vi "LabVIEW_MQTT_Toolkit_V2.vi"() -> ()   [LabVIEW 2021] (continued)
                  n1492 = Format Date/Time String(seconds (now)=w3662, UTC format=TRUE) -> (date/time string=w3664:string)  [unwired: 1 in]
                  n1493 = Build Array(w3677, w3680) -> (w3679:string[])
                  n1494 = Scan From String(format string="%<%x %H:%M:%S%3u>T", input string=w3664) -> (output 1=w3665:timestamp)  [unwired: 3 in, 3 out]
                  n1495 = To Double Precision Float(number=w3665) -> (double precision float=w3663:dbl)
                }
                n1496 = Concatenate Strings(w3623, "TimeStamp;MeasureCh_Z(g);", "\n") -> (w3639:string)
                n1497 = Build Path(base path=w3640, name or relative path="Logfile") -> (appended path=w3641:path)
                n1498 = Search and Replace String(replace all?=TRUE ("replace all? (F)"), input string=w3634, search string="/") -> (result string=w3646:string)  [unwired: 5 in, 3 out]
                n1499 = call <vilib>:"Check if File or Folder Exists.vi"("path"=w3641) -> ("file or folder exists?"=w3642:bool, "dup path"=w3643:path)  [unwired: 8 in, 1 out]
                n1500 = case shown="False" w3642 {
                  tunnel: w3643 -> [w3660 w3661]
                  tunnel: [w3659 w3661] -> w3644
                  frame False {
                    n1501 = Create Folder(path (use dialog)=w3660) -> (created path=w3659:path)  [unwired: 2 in, 2 out]
                  }
                  frame True {
                  }
                }
                n1502 = Concatenate Strings(w3646, "_" ("string"), "S_E_T.csv") -> (w3647:string)
                n1503 = Build Path(base path=w3644, name or relative path=w3647) -> (appended path=w3645:path)
                n1504 = Open/Create/Replace File(file path (use dialog)=w3645, operation (0:open)=T11."open or create") -> (refnum out=w3638:refnum<file>, error out=w3636:errorcluster)  [unwired: 4 in, 1 out]
                n1505 = Write to Text File(file (use dialog)=w3638, text=w3639, error in=w3636) -> (refnum out=w3637:refnum<file>, error out=w3635:errorcluster)  [unwired: 1 in, 1 out]
                n1506 = Close File(refnum=w3637, error in=w3635) -> (path=w3624:path)  [unwired: 1 out]
              }
              frame 2 {
                w3689 = T14 2 items=["User Home"=0, "User Desktop"=1, "User Documents"=2, "User Application Data"=3, "User Preferences"=4, "User Temporary"=5, "Public Documents"=6, "Public Application Data"=7, "Public Preferences"=8, "Public Cache"=13, "System Core Libraries"=9, "System Installed Libraries"=10, "Application Files"=11, "Boot Volume Root"=12] ("system directory type")
                n1507 = Decimate 1D Array(w3716) -> (w3714:dbl[])
                n1508 = Search and Replace String(replace all?=TRUE ("replace all? (F)"), input string=w3684, search string="/") -> (result string=w3705:string)  [unwired: 5 in, 3 out]
                n1509 = for {
                  tunnel: w3714 -> [w3735] mode=indexing
                  tunnel: [w3738] -> w3713 mode=indexing
                  tunnel: w3715 -> [w3737] mode=indexing
                  tunnel: [w3735] -> w3712 mode=indexing
                  tunnel: w3711 -> [w3730]
                  tunnel: w3710 -> [w3729]
                  tunnel: w3709 -> [w3728] mode=indexing
                  tunnel: w3708 -> [w3727]
                  tunnel: [w3722] -> w3707
                  n1510 = Join Numbers(hi=w3730, lo=w3729) -> ((hi.lo)=w3732:u32)
                  n1511 = To Double Precision Float(number=w3728) -> (double precision float=w3733:dbl)
                  n1512 = Number To Decimal String(number=w3737) -> (decimal integer string=w3736:string)  [unwired: 1 in]
                  n1513 = Number To Fractional String(number=w3735, precision (6)=i16 3 ("width (-)")) -> (F-format string=w3739:string)  [unwired: 2 in]
                  n1514 = Divide(x=w3733, y=w3727) -> (x/y=w3734:dbl)
                  n1515 = Build Array(w3736, w3739) -> (w3738:string[])
                  n1516 = To Unsigned Quad Integer(1:w3732) -> (0:w3731:u64)
                  n1517 = call "Unix Time to Timestamp.vi"("Fractional Second"=w3734, "Unix Time (s)"=w3731) -> ("Timestamp"=w3721:timestamp)  [unwired: 8 in, 1 out]
                  n1518 = Format Date/Time String(seconds (now)=w3721, UTC format=TRUE) -> (date/time string=w3723:string)  [unwired: 1 in]
                  n1519 = Scan From String(format string="%<%x %H:%M:%S%3u>T", input string=w3723) -> (output 1=w3724:timestamp)  [unwired: 3 in, 3 out]
                  n1520 = To Double Precision Float(number=w3724) -> (double precision float=w3722:dbl)
                }
                n1521 = Concatenate Strings(w3682, "TimeStamp;MeasureCh_X(g);", "\n") -> (w3698:string)
                n1522 = Concatenate Strings(w3705, "_" ("string"), "S_E_T.csv") -> (w3706:string)
                n1523 = call <vilib>:"Get System Directory.vi"("system directory type"=w3689) -> ("system directory"=w3699:path)  [unwired: 10 in]
                n1524 = Build Path(base path=w3699, name or relative path="Logfile") -> (appended path=w3700:path)
                n1525 = call <vilib>:"Check if File or Folder Exists.vi"("path"=w3700) -> ("file or folder exists?"=w3701:bool, "dup path"=w3702:path)  [unwired: 8 in, 1 out]
                n1526 = case shown="False" w3701 {
                  tunnel: w3702 -> [w3719 w3720]
                  tunnel: [w3718 w3720] -> w3703
                  frame False {
                    n1527 = Create Folder(path (use dialog)=w3719) -> (created path=w3718:path)  [unwired: 2 in, 2 out]
                  }
                  frame True {
                  }
                }
                n1528 = Build Path(base path=w3703, name or relative path=w3706) -> (appended path=w3704:path)
                n1529 = Open/Create/Replace File(file path (use dialog)=w3704, operation (0:open)=T11."open or create") -> (refnum out=w3697:refnum<file>, error out=w3695:errorcluster)  [unwired: 4 in, 1 out]
                n1530 = Write to Text File(file (use dialog)=w3697, text=w3698, error in=w3695) -> (refnum out=w3696:refnum<file>, error out=w3694:errorcluster)  [unwired: 1 in, 1 out]
                n1531 = Close File(refnum=w3696, error in=w3694) -> (path=w3683:path)  [unwired: 1 out]
              }
              frame 3 {
                w3748 = T14 2 items=["User Home"=0, "User Desktop"=1, "User Documents"=2, "User Application Data"=3, "User Preferences"=4, "User Temporary"=5, "Public Documents"=6, "Public Application Data"=7, "Public Preferences"=8, "Public Cache"=13, "System Core Libraries"=9, "System Installed Libraries"=10, "Application Files"=11, "Boot Volume Root"=12] ("system directory type")
                n1532 = Decimate 1D Array(w3777) -> (w3775:dbl[], w3774:dbl[])
                n1533 = Search and Replace String(replace all?=TRUE ("replace all? (F)"), input string=w3743, search string="/") -> (result string=w3764:string)  [unwired: 5 in, 3 out]
                n1534 = Concatenate Strings(w3741, "TimeStamp;MeasureCh_Z(g);Ch_X(g);", "\n") -> (w3757:string)
                n1535 = for {
                  tunnel: w3775 -> [w3797] mode=indexing
                  tunnel: w3774 -> [w3796] mode=indexing
                  tunnel: [w3800] -> w3773 mode=indexing
                  tunnel: w3776 -> [w3799] mode=indexing
                  tunnel: [w3797] -> w3772 mode=indexing
                  tunnel: [w3796] -> w3771 mode=indexing
                  tunnel: w3770 -> [w3791]
                  tunnel: w3769 -> [w3790]
                  tunnel: w3768 -> [w3789] mode=indexing
                  tunnel: w3767 -> [w3788]
                  tunnel: [w3783] -> w3766
                  n1536 = Join Numbers(hi=w3791, lo=w3790) -> ((hi.lo)=w3793:u32)
                  n1537 = To Double Precision Float(number=w3789) -> (double precision float=w3794:dbl)
                  n1538 = Number To Decimal String(number=w3799) -> (decimal integer string=w3798:string)  [unwired: 1 in]
                  n1539 = Number To Fractional String(number=w3797, precision (6)=i16 3 ("width (-)")) -> (F-format string=w3802:string)  [unwired: 2 in]
                  n1540 = Number To Fractional String(number=w3796, precision (6)=i16 3 ("width (-)")) -> (F-format string=w3801:string)  [unwired: 2 in]
                  n1541 = Divide(x=w3794, y=w3788) -> (x/y=w3795:dbl)
                  n1542 = Build Array(w3798, w3802, w3801) -> (w3800:string[])
                  n1543 = To Unsigned Quad Integer(1:w3793) -> (0:w3792:u64)
                  n1544 = call "Unix Time to Timestamp.vi"("Fractional Second"=w3795, "Unix Time (s)"=w3792) -> ("Timestamp"=w3782:timestamp)  [unwired: 8 in, 1 out]
                  n1545 = Format Date/Time String(seconds (now)=w3782, UTC format=TRUE) -> (date/time string=w3784:string)  [unwired: 1 in]
                  n1546 = Scan From String(format string="%<%x %H:%M:%S%3u>T", input string=w3784) -> (output 1=w3785:timestamp)  [unwired: 3 in, 3 out]
                  n1547 = To Double Precision Float(number=w3785) -> (double precision float=w3783:dbl)
                }
                n1548 = Concatenate Strings(w3764, "_" ("string"), "S_E_T.csv") -> (w3765:string)
                n1549 = call <vilib>:"Get System Directory.vi"("system directory type"=w3748) -> ("system directory"=w3758:path)  [unwired: 10 in]
                n1550 = Build Path(base path=w3758, name or relative path="Logfile") -> (appended path=w3759:path)
                n1551 = call <vilib>:"Check if File or Folder Exists.vi"("path"=w3759) -> ("file or folder exists?"=w3760:bool, "dup path"=w3761:path)  [unwired: 8 in, 1 out]
                n1552 = case shown="False" w3760 {
                  tunnel: w3761 -> [w3780 w3781]
                  tunnel: [w3779 w3781] -> w3762
                  frame False {
                    n1553 = Create Folder(path (use dialog)=w3780) -> (created path=w3779:path)  [unwired: 2 in, 2 out]
                  }
                  frame True {
                  }
                }
                n1554 = Build Path(base path=w3762, name or relative path=w3765) -> (appended path=w3763:path)
                n1555 = Open/Create/Replace File(file path (use dialog)=w3763, operation (0:open)=T11."open or create") -> (refnum out=w3756:refnum<file>, error out=w3754:errorcluster)  [unwired: 4 in, 1 out]
                n1556 = Write to Text File(file (use dialog)=w3756, text=w3757, error in=w3754) -> (refnum out=w3755:refnum<file>, error out=w3753:errorcluster)  [unwired: 1 in, 1 out]
                n1557 = Close File(refnum=w3755, error in=w3753) -> (path=w3742:path)  [unwired: 1 out]
              }
              frame 4 {
                w3812 = T14 2 items=["User Home"=0, "User Desktop"=1, "User Documents"=2, "User Application Data"=3, "User Preferences"=4, "User Temporary"=5, "Public Documents"=6, "Public Application Data"=7, "Public Preferences"=8, "Public Cache"=13, "System Core Libraries"=9, "System Installed Libraries"=10, "Application Files"=11, "Boot Volume Root"=12] ("system directory type")
                # "this function calculate Time  of subpacket"
                n1558 = Decimate 1D Array(w3839) -> (w3838:dbl[])
                n1559 = Search and Replace String(replace all?=TRUE ("replace all? (F)"), input string=w3807, search string="/") -> (result string=w3828:string)  [unwired: 5 in, 3 out]
                n1560 = Concatenate Strings(w3805, "TimeStamp;MeasureCh_Y(g);", "\n") -> (w3821:string)
                n1561 = for {
                  tunnel: w3838 -> [w3858] mode=indexing
                  tunnel: [w3861] -> w3836 mode=indexing
                  tunnel: w3837 -> [w3860] mode=indexing
                  tunnel: [w3858] -> w3835 mode=indexing
                  tunnel: w3834 -> [w3853]
                  tunnel: w3833 -> [w3850]
                  tunnel: w3832 -> [w3851] mode=indexing
                  tunnel: w3831 -> [w3852]
                  tunnel: [w3844] -> w3830
                  n1562 = Join Numbers(hi=w3853, lo=w3850) -> ((hi.lo)=w3855:u32)
                  n1563 = To Double Precision Float(number=w3851) -> (double precision float=w3856:dbl)
                  n1564 = Number To Decimal String(number=w3860) -> (decimal integer string=w3859:string)  [unwired: 1 in]
                  n1565 = Number To Fractional String(number=w3858, precision (6)=i16 3 ("width (-)")) -> (F-format string=w3862:string)  [unwired: 2 in]
                  n1566 = Divide(x=w3856, y=w3852) -> (x/y=w3857:dbl)
                  n1567 = Build Array(w3859, w3862) -> (w3861:string[])
                  n1568 = To Unsigned Quad Integer(1:w3855) -> (0:w3854:u64)
                  n1569 = call "Unix Time to Timestamp.vi"("Fractional Second"=w3857, "Unix Time (s)"=w3854) -> ("Timestamp"=w3845:timestamp)  [unwired: 8 in, 1 out]
                  n1570 = Format Date/Time String(seconds (now)=w3845, UTC format=TRUE) -> (date/time string=w3846:string)  [unwired: 1 in]
                  n1571 = Scan From String(format string="%<%x %H:%M:%S%3u>T", input string=w3846) -> (output 1=w3847:timestamp)  [unwired: 3 in, 3 out]
                  n1572 = To Double Precision Float(number=w3847) -> (double precision float=w3844:dbl)
                }
                n1573 = Concatenate Strings(w3828, "_" ("string"), "S_E_T.csv") -> (w3829:string)
                n1574 = call <vilib>:"Get System Directory.vi"("system directory type"=w3812) -> ("system directory"=w3822:path)  [unwired: 10 in]
                n1575 = Build Path(base path=w3822, name or relative path="Logfile") -> (appended path=w3823:path)
                n1576 = call <vilib>:"Check if File or Folder Exists.vi"("path"=w3823) -> ("file or folder exists?"=w3824:bool, "dup path"=w3825:path)  [unwired: 8 in, 1 out]
                n1577 = case shown="False" w3824 {
                  tunnel: w3825 -> [w3842 w3843]
                  tunnel: [w3841 w3843] -> w3826
                  frame False {
                    n1578 = Create Folder(path (use dialog)=w3842) -> (created path=w3841:path)  [unwired: 2 in, 2 out]
                  }
                  frame True {
                  }
                }
                n1579 = Build Path(base path=w3826, name or relative path=w3829) -> (appended path=w3827:path)
                n1580 = Open/Create/Replace File(file path (use dialog)=w3827, operation (0:open)=T11."open or create") -> (refnum out=w3820:refnum<file>, error out=w3818:errorcluster)  [unwired: 4 in, 1 out]
                n1581 = Write to Text File(file (use dialog)=w3820, text=w3821, error in=w3818) -> (refnum out=w3819:refnum<file>, error out=w3817:errorcluster)  [unwired: 1 in, 1 out]
                n1582 = Close File(refnum=w3819, error in=w3817) -> (path=w3806:path)  [unwired: 1 out]
              }
              frame 5 {
                w3871 = T14 2 items=["User Home"=0, "User Desktop"=1, "User Documents"=2, "User Application Data"=3, "User Preferences"=4, "User Temporary"=5, "Public Documents"=6, "Public Application Data"=7, "Public Preferences"=8, "Public Cache"=13, "System Core Libraries"=9, "System Installed Libraries"=10, "Application Files"=11, "Boot Volume Root"=12] ("system directory type")
                n1583 = Decimate 1D Array(w3901) -> (w3897:dbl[], w3898:dbl[])
                n1584 = Search and Replace String(replace all?=TRUE ("replace all? (F)"), input string=w3865, search string="/") -> (result string=w3887:string)  [unwired: 5 in, 3 out]
                n1585 = for {
                  tunnel: [w3924] -> w3899 mode=indexing
                  tunnel: w3900 -> [w3923] mode=indexing
                  tunnel: w3897 -> [w3921] mode=indexing
                  tunnel: w3898 -> [w3920] mode=indexing
                  tunnel: [w3921] -> w3896 mode=indexing
                  tunnel: [w3920] -> w3895 mode=indexing
                  tunnel: w3894 -> [w3915]
                  tunnel: w3893 -> [w3914]
                  tunnel: w3892 -> [w3913] mode=indexing
                  tunnel: w3891 -> [w3912]
                  tunnel: [w3907] -> w3890
                  tunnel: [w3907] -> w3889
                  n1586 = Join Numbers(hi=w3915, lo=w3914) -> ((hi.lo)=w3917:u32)
                  n1587 = To Double Precision Float(number=w3913) -> (double precision float=w3918:dbl)
                  n1588 = Number To Decimal String(number=w3923) -> (decimal integer string=w3922:string)  [unwired: 1 in]
                  n1589 = Number To Fractional String(number=w3921, precision (6)=i16 3 ("width (-)")) -> (F-format string=w3926:string)  [unwired: 2 in]
                  n1590 = Number To Fractional String(number=w3920, precision (6)=i16 3 ("width (-)")) -> (F-format string=w3925:string)  [unwired: 2 in]
                  n1591 = Divide(x=w3918, y=w3912) -> (x/y=w3919:dbl)
                  n1592 = Build Array(w3922, w3926, w3925) -> (w3924:string[])
                  n1593 = To Unsigned Quad Integer(1:w3917) -> (0:w3916:u64)
                  n1594 = call "Unix Time to Timestamp.vi"("Fractional Second"=w3919, "Unix Time (s)"=w3916) -> ("Timestamp"=w3906:timestamp)  [unwired: 8 in, 1 out]
                  n1595 = Format Date/Time String(seconds (now)=w3906, UTC format=TRUE) -> (date/time string=w3908:string)  [unwired: 1 in]
                  n1596 = Scan From String(format string="%<%x %H:%M:%S%3u>T", input string=w3908) -> (output 1=w3909:timestamp)  [unwired: 3 in, 3 out]
                  n1597 = To Double Precision Float(number=w3909) -> (double precision float=w3907:dbl)
                }
                n1598 = Concatenate Strings(w3864, "TimeStamp;MeasureCh_Z(g);Ch_Y(g);", "\n") -> (w3880:string)
                n1599 = Concatenate Strings(w3887, "_" ("string"), "S_E_T.csv") -> (w3888:string)
                n1600 = call <vilib>:"Get System Directory.vi"("system directory type"=w3871) -> ("system directory"=w3881:path)  [unwired: 10 in]
                n1601 = Build Path(base path=w3881, name or relative path="Logfile") -> (appended path=w3882:path)
                n1602 = call <vilib>:"Check if File or Folder Exists.vi"("path"=w3882) -> ("file or folder exists?"=w3883:bool, "dup path"=w3884:path)  [unwired: 8 in, 1 out]
                n1603 = case shown="False" w3883 {
                  tunnel: w3884 -> [w3904 w3905]
                  tunnel: [w3903 w3905] -> w3885
                  frame False {
                    n1604 = Create Folder(path (use dialog)=w3904) -> (created path=w3903:path)  [unwired: 2 in, 2 out]
                  }
                  frame True {
                  }
                }
                n1605 = Build Path(base path=w3885, name or relative path=w3888) -> (appended path=w3886:path)
                n1606 = Open/Create/Replace File(file path (use dialog)=w3886, operation (0:open)=T11."open or create") -> (refnum out=w3879:refnum<file>, error out=w3877:errorcluster)  [unwired: 4 in, 1 out]
                n1607 = Write to Text File(file (use dialog)=w3879, text=w3880, error in=w3877) -> (refnum out=w3878:refnum<file>, error out=w3876:errorcluster)  [unwired: 1 in, 1 out]
                n1608 = Close File(refnum=w3878, error in=w3876) -> (path=w3866:path)  [unwired: 1 out]
              }
              frame 6 {
                w3936 = T14 2 items=["User Home"=0, "User Desktop"=1, "User Documents"=2, "User Application Data"=3, "User Preferences"=4, "User Temporary"=5, "Public Documents"=6, "Public Application Data"=7, "Public Preferences"=8, "Public Cache"=13, "System Core Libraries"=9, "System Installed Libraries"=10, "Application Files"=11, "Boot Volume Root"=12] ("system directory type")
                n1609 = Decimate 1D Array(w3966) -> (w3964:dbl[], w3963:dbl[])
                n1610 = Search and Replace String(replace all?=TRUE ("replace all? (F)"), input string=w3931, search string="/") -> (result string=w3952:string)  [unwired: 5 in, 3 out]
                n1611 = for {
                  tunnel: w3964 -> [w3986] mode=indexing
                  tunnel: w3963 -> [w3985] mode=indexing
                  tunnel: [w3989] -> w3962 mode=indexing
                  tunnel: w3965 -> [w3988] mode=indexing
                  tunnel: [w3986] -> w3961 mode=indexing
                  tunnel: [w3985] -> w3960 mode=indexing
                  tunnel: w3959 -> [w3980]
                  tunnel: w3958 -> [w3979]
                  tunnel: w3957 -> [w3978] mode=indexing
                  tunnel: w3956 -> [w3977]
                  tunnel: [w3972] -> w3955
                  tunnel: [w3972] -> w3954
                  n1612 = Join Numbers(hi=w3980, lo=w3979) -> ((hi.lo)=w3982:u32)
                  n1613 = To Double Precision Float(number=w3978) -> (double precision float=w3983:dbl)
                  n1614 = Number To Decimal String(number=w3988) -> (decimal integer string=w3987:string)  [unwired: 1 in]
                  n1615 = Number To Fractional String(number=w3986, precision (6)=i16 3 ("width (-)")) -> (F-format string=w3991:string)  [unwired: 2 in]
                  n1616 = Number To Fractional String(number=w3985, precision (6)=i16 3 ("width (-)")) -> (F-format string=w3990:string)  [unwired: 2 in]
                  n1617 = Divide(x=w3983, y=w3977) -> (x/y=w3984:dbl)
                  n1618 = Build Array(w3987, w3991, w3990) -> (w3989:string[])
                  n1619 = To Unsigned Quad Integer(1:w3982) -> (0:w3981:u64)
                  n1620 = call "Unix Time to Timestamp.vi"("Fractional Second"=w3984, "Unix Time (s)"=w3981) -> ("Timestamp"=w3971:timestamp)  [unwired: 8 in, 1 out]
                  n1621 = Format Date/Time String(seconds (now)=w3971, UTC format=TRUE) -> (date/time string=w3973:string)  [unwired: 1 in]
                  n1622 = Scan From String(format string="%<%x %H:%M:%S%3u>T", input string=w3973) -> (output 1=w3974:timestamp)  [unwired: 3 in, 3 out]
                  n1623 = To Double Precision Float(number=w3974) -> (double precision float=w3972:dbl)
                }
                n1624 = Concatenate Strings(w3930, "TimeStamp;MeasureCh_X(g);Ch_Y(g);", "\n") -> (w3945:string)
                n1625 = Concatenate Strings(w3952, "_" ("string"), "S_E_T.csv") -> (w3953:string)
                n1626 = call <vilib>:"Get System Directory.vi"("system directory type"=w3936) -> ("system directory"=w3946:path)  [unwired: 10 in]
                n1627 = Build Path(base path=w3946, name or relative path="Logfile") -> (appended path=w3947:path)
                n1628 = call <vilib>:"Check if File or Folder Exists.vi"("path"=w3947) -> ("file or folder exists?"=w3948:bool, "dup path"=w3949:path)  [unwired: 8 in, 1 out]
                n1629 = case shown="False" w3948 {
                  tunnel: w3949 -> [w3969 w3970]
                  tunnel: [w3968 w3970] -> w3950
                  frame False {
                    n1630 = Create Folder(path (use dialog)=w3969) -> (created path=w3968:path)  [unwired: 2 in, 2 out]
                  }
                  frame True {
                  }
                }
                n1631 = Build Path(base path=w3950, name or relative path=w3953) -> (appended path=w3951:path)
                n1632 = Open/Create/Replace File(file path (use dialog)=w3951, operation (0:open)=T11."open or create") -> (refnum out=w3944:refnum<file>, error out=w3942:errorcluster)  [unwired: 4 in, 1 out]
                n1633 = Write to Text File(file (use dialog)=w3944, text=w3945, error in=w3942) -> (refnum out=w3943:refnum<file>, error out=w3941:errorcluster)  [unwired: 1 in, 1 out]
                n1634 = Close File(refnum=w3943, error in=w3941) -> (path=w3929:path)  [unwired: 1 out]
              }
              frame 7 {
                w4001 = T14 2 items=["User Home"=0, "User Desktop"=1, "User Documents"=2, "User Application Data"=3, "User Preferences"=4, "User Temporary"=5, "Public Documents"=6, "Public Application Data"=7, "Public Preferences"=8, "Public Cache"=13, "System Core Libraries"=9, "System Installed Libraries"=10, "Application Files"=11, "Boot Volume Root"=12] ("system directory type")
                n1635 = Search and Replace String(replace all?=TRUE ("replace all? (F)"), input string=w3996, search string="/") -> (result string=w4017:string)  [unwired: 5 in, 3 out]
                n1636 = Concatenate Strings(w3994, "TimeStamp;MeasureCh_Z(g);Ch_X(g);Ch_Y(g);", "\n") -> (w4010:string)
                n1637 = Concatenate Strings(w4017, "_" ("string"), "S_E_T.csv") -> (w4018:string)
                n1638 = call <vilib>:"Get System Directory.vi"("system directory type"=w4001) -> ("system directory"=w4011:path)  [unwired: 10 in]
                n1639 = Decimate 1D Array(w4034) -> (w4033:dbl[], w4032:dbl[], w4031:dbl[])
                n1640 = for {
                  tunnel: w4033 -> [w4055] mode=indexing
                  tunnel: w4032 -> [w4054] mode=indexing
                  tunnel: w4031 -> [w4053] mode=indexing
                  tunnel: [w4058] -> w4030 mode=indexing
                  tunnel: w4029 -> [w4057] mode=indexing
                  tunnel: [w4055] -> w4028 mode=indexing
                  tunnel: [w4054] -> w4027 mode=indexing
                  tunnel: [w4053] -> w4026 mode=indexing
                  tunnel: w4025 -> [w4048]
                  tunnel: w4024 -> [w4047]
                  tunnel: w4023 -> [w4046] mode=indexing
                  tunnel: w4022 -> [w4045]
                  tunnel: [w4039] -> w4021
                  tunnel: [w4039] -> w4020
                  tunnel: [w4039] -> w4019
                  n1641 = Join Numbers(hi=w4048, lo=w4047) -> ((hi.lo)=w4050:u32)
                  n1642 = To Double Precision Float(number=w4046) -> (double precision float=w4051:dbl)
                  n1643 = Number To Decimal String(number=w4057) -> (decimal integer string=w4056:string)  [unwired: 1 in]
                  n1644 = Number To Fractional String(number=w4055, precision (6)=i16 3 ("width (-)")) -> (F-format string=w4062:string)  [unwired: 2 in]
                  n1645 = Number To Fractional String(number=w4054, precision (6)=i16 3 ("width (-)")) -> (F-format string=w4061:string)  [unwired: 2 in]
                  n1646 = Number To Fractional String(number=w4053, precision (6)=i16 3 ("width (-)")) -> (F-format string=w4059:string)  [unwired: 2 in]
                  n1647 = Build Array(w4056, w4062, w4061, w4059) -> (w4058:string[])
                  n1648 = Divide(x=w4051, y=w4045) -> (x/y=w4052:dbl)
                  n1649 = To Unsigned Quad Integer(1:w4050) -> (0:w4049:u64)
                  n1650 = call "Unix Time to Timestamp.vi"("Fractional Second"=w4052, "Unix Time (s)"=w4049) -> ("Timestamp"=w4040:timestamp)  [unwired: 8 in, 1 out]
                  n1651 = Format Date/Time String(seconds (now)=w4040, UTC format=TRUE) -> (date/time string=w4041:string)  [unwired: 1 in]
                  n1652 = Scan From String(format string="%<%x %H:%M:%S%3u>T", input string=w4041) -> (output 1=w4042:timestamp)  [unwired: 3 in, 3 out]
                  n1653 = To Double Precision Float(number=w4042) -> (double precision float=w4039:dbl)
                }
                n1654 = Build Path(base path=w4011, name or relative path="Logfile") -> (appended path=w4012:path)
                n1655 = call <vilib>:"Check if File or Folder Exists.vi"("path"=w4012) -> ("file or folder exists?"=w4013:bool, "dup path"=w4014:path)  [unwired: 8 in, 1 out]
                n1656 = case shown="False" w4013 {
                  tunnel: w4014 -> [w4037 w4038]
                  tunnel: [w4036 w4038] -> w4015
                  frame False {
                    n1657 = Create Folder(path (use dialog)=w4037) -> (created path=w4036:path)  [unwired: 2 in, 2 out]
                  }
                  frame True {
                  }
                }
                n1658 = Build Path(base path=w4015, name or relative path=w4018) -> (appended path=w4016:path)
                n1659 = Open/Create/Replace File(file path (use dialog)=w4016, operation (0:open)=T11."open or create") -> (refnum out=w4009:refnum<file>, error out=w4007:errorcluster)  [unwired: 4 in, 1 out]
                n1660 = Write to Text File(file (use dialog)=w4009, text=w4010, error in=w4007) -> (refnum out=w4008:refnum<file>, error out=w4006:errorcluster)  [unwired: 1 in, 1 out]
                n1661 = Close File(refnum=w4008, error in=w4006) -> (path=w3995:path)  [unwired: 1 out]
              }
              frame 8 {
                w4072 = T14 2 items=["User Home"=0, "User Desktop"=1, "User Documents"=2, "User Application Data"=3, "User Preferences"=4, "User Temporary"=5, "Public Documents"=6, "Public Application Data"=7, "Public Preferences"=8, "Public Cache"=13, "System Core Libraries"=9, "System Installed Libraries"=10, "Application Files"=11, "Boot Volume Root"=12] ("system directory type")
                n1662 = Decimate 1D Array(w4099) -> (w4096:dbl[])
                n1663 = Search and Replace String(replace all?=TRUE ("replace all? (F)"), input string=w4067, search string="/") -> (result string=w4088:string)  [unwired: 5 in, 3 out]
                n1664 = for {
                  tunnel: [w4122] -> w4098 mode=indexing
                  tunnel: w4097 -> [w4119] mode=indexing
                  tunnel: w4096 -> [w4118] mode=indexing
                  tunnel: [w4118] -> w4095 mode=indexing
                  tunnel: w4094 -> [w4113]
                  tunnel: w4093 -> [w4112]
                  tunnel: w4092 -> [w4111] mode=indexing
                  tunnel: w4091 -> [w4110]
                  tunnel: [w4104] -> w4090
                  n1665 = Join Numbers(hi=w4113, lo=w4112) -> ((hi.lo)=w4115:u32)
                  n1666 = To Double Precision Float(number=w4111) -> (double precision float=w4116:dbl)
                  n1667 = Number To Decimal String(number=w4119) -> (decimal integer string=w4121:string)  [unwired: 1 in]
                  n1668 = Number To Fractional String(number=w4118, precision (6)=i16 3 ("width (-)")) -> (F-format string=w4120:string)  [unwired: 2 in]
                  n1669 = Divide(x=w4116, y=w4110) -> (x/y=w4117:dbl)
                  n1670 = Build Array(w4121, w4120) -> (w4122:string[])
                  n1671 = To Unsigned Quad Integer(1:w4115) -> (0:w4114:u64)
                  n1672 = call "Unix Time to Timestamp.vi"("Fractional Second"=w4117, "Unix Time (s)"=w4114) -> ("Timestamp"=w4105:timestamp)  [unwired: 8 in, 1 out]
                  n1673 = Format Date/Time String(seconds (now)=w4105, UTC format=TRUE) -> (date/time string=w4106:string)  [unwired: 1 in]
                  n1674 = Scan From String(format string="%<%x %H:%M:%S%3u>T", input string=w4106) -> (output 1=w4107:timestamp)  [unwired: 3 in, 3 out]
                  n1675 = To Double Precision Float(number=w4107) -> (double precision float=w4104:dbl)
                }
                n1676 = Concatenate Strings(w4065, "TimeStamp;Measure INC_X(Deg);", "\n") -> (w4081:string)
                n1677 = Concatenate Strings(w4088, "_" ("string"), "S_E_T.csv") -> (w4089:string)
                n1678 = call <vilib>:"Get System Directory.vi"("system directory type"=w4072) -> ("system directory"=w4082:path)  [unwired: 10 in]
                n1679 = Build Path(base path=w4082, name or relative path="Logfile") -> (appended path=w4083:path)
                n1680 = call <vilib>:"Check if File or Folder Exists.vi"("path"=w4083) -> ("file or folder exists?"=w4084:bool, "dup path"=w4085:path)  [unwired: 8 in, 1 out]
                n1681 = case shown="False" w4084 {
                  tunnel: w4085 -> [w4102 w4103]
                  tunnel: [w4101 w4103] -> w4086
                  frame False {
                    n1682 = Create Folder(path (use dialog)=w4102) -> (created path=w4101:path)  [unwired: 2 in, 2 out]
                  }
                  frame True {
                  }
                }
                n1683 = Build Path(base path=w4086, name or relative path=w4089) -> (appended path=w4087:path)
                n1684 = Open/Create/Replace File(file path (use dialog)=w4087, operation (0:open)=T11."open or create") -> (refnum out=w4080:refnum<file>, error out=w4078:errorcluster)  [unwired: 4 in, 1 out]
                n1685 = Write to Text File(file (use dialog)=w4080, text=w4081, error in=w4078) -> (refnum out=w4079:refnum<file>, error out=w4077:errorcluster)  [unwired: 1 in, 1 out]
                n1686 = Close File(refnum=w4079, error in=w4077) -> (path=w4066:path)  [unwired: 1 out]
              }
              frame 9 {
                w4131 = T14 2 items=["User Home"=0, "User Desktop"=1, "User Documents"=2, "User Application Data"=3, "User Preferences"=4, "User Temporary"=5, "Public Documents"=6, "Public Application Data"=7, "Public Preferences"=8, "Public Cache"=13, "System Core Libraries"=9, "System Installed Libraries"=10, "Application Files"=11, "Boot Volume Root"=12] ("system directory type")
                n1687 = Decimate 1D Array(w4161) -> (w4157:dbl[], w4160:dbl[])
                n1688 = Search and Replace String(replace all?=TRUE ("replace all? (F)"), input string=w4126, search string="/") -> (result string=w4147:string)  [unwired: 5 in, 3 out]
                n1689 = for {
                  tunnel: [w4184] -> w4158 mode=indexing
                  tunnel: w4157 -> [w4181] mode=indexing
                  tunnel: w4160 -> [w4180] mode=indexing
                  tunnel: w4159 -> [w4182] mode=indexing
                  tunnel: [w4181] -> w4156 mode=indexing
                  tunnel: [w4180] -> w4155 mode=indexing
                  tunnel: w4154 -> [w4175]
                  tunnel: w4153 -> [w4174]
                  tunnel: w4152 -> [w4173] mode=indexing
                  tunnel: w4151 -> [w4172]
                  tunnel: [w4166] -> w4149
                  tunnel: [w4166] -> w4150
                  n1690 = Join Numbers(hi=w4175, lo=w4174) -> ((hi.lo)=w4177:u32)
                  n1691 = To Double Precision Float(number=w4173) -> (double precision float=w4178:dbl)
                  n1692 = Number To Decimal String(number=w4182) -> (decimal integer string=w4183:string)  [unwired: 1 in]
                  n1693 = Number To Fractional String(number=w4181, precision (6)=i16 3 ("width (-)")) -> (F-format string=w4186:string)  [unwired: 2 in]
                  n1694 = Number To Fractional String(number=w4180, precision (6)=i16 3 ("width (-)")) -> (F-format string=w4185:string)  [unwired: 2 in]
                  n1695 = Divide(x=w4178, y=w4172) -> (x/y=w4179:dbl)
                  n1696 = Build Array(w4183, w4186, w4185) -> (w4184:string[])
                  n1697 = To Unsigned Quad Integer(1:w4177) -> (0:w4176:u64)
                  n1698 = call "Unix Time to Timestamp.vi"("Fractional Second"=w4179, "Unix Time (s)"=w4176) -> ("Timestamp"=w4167:timestamp)  [unwired: 8 in, 1 out]
                  n1699 = Format Date/Time String(seconds (now)=w4167, UTC format=TRUE) -> (date/time string=w4168:string)  [unwired: 1 in]
                  n1700 = Scan From String(format string="%<%x %H:%M:%S%3u>T", input string=w4168) -> (output 1=w4169:timestamp)  [unwired: 3 in, 3 out]
                  n1701 = To Double Precision Float(number=w4169) -> (double precision float=w4166:dbl)
                }
                n1702 = Concatenate Strings(w4124, "TimeStamp;Measure Ch_Z(g);INC_X(Deg);", "\n") -> (w4140:string)
                n1703 = Concatenate Strings(w4147, "_" ("string"), "S_E_T.csv") -> (w4148:string)
                n1704 = call <vilib>:"Get System Directory.vi"("system directory type"=w4131) -> ("system directory"=w4141:path)  [unwired: 10 in]
                n1705 = Build Path(base path=w4141, name or relative path="Logfile") -> (appended path=w4142:path)
                n1706 = call <vilib>:"Check if File or Folder Exists.vi"("path"=w4142) -> ("file or folder exists?"=w4143:bool, "dup path"=w4144:path)  [unwired: 8 in, 1 out]
                n1707 = case shown="False" w4143 {
                  tunnel: w4144 -> [w4164 w4165]
                  tunnel: [w4163 w4165] -> w4145
                  frame False {
                    n1708 = Create Folder(path (use dialog)=w4164) -> (created path=w4163:path)  [unwired: 2 in, 2 out]
                  }
                  frame True {
                  }
                }
                n1709 = Build Path(base path=w4145, name or relative path=w4148) -> (appended path=w4146:path)
                n1710 = Open/Create/Replace File(file path (use dialog)=w4146, operation (0:open)=T11."open or create") -> (refnum out=w4139:refnum<file>, error out=w4137:errorcluster)  [unwired: 4 in, 1 out]
                n1711 = Write to Text File(file (use dialog)=w4139, text=w4140, error in=w4137) -> (refnum out=w4138:refnum<file>, error out=w4136:errorcluster)  [unwired: 1 in, 1 out]
                n1712 = Close File(refnum=w4138, error in=w4136) -> (path=w4125:path)  [unwired: 1 out]
              }
              frame 10 {
                w4196 = T14 2 items=["User Home"=0, "User Desktop"=1, "User Documents"=2, "User Application Data"=3, "User Preferences"=4, "User Temporary"=5, "Public Documents"=6, "Public Application Data"=7, "Public Preferences"=8, "Public Cache"=13, "System Core Libraries"=9, "System Installed Libraries"=10, "Application Files"=11, "Boot Volume Root"=12] ("system directory type")
                n1713 = Decimate 1D Array(w4226) -> (w4223:dbl[], w4222:dbl[])
                n1714 = Search and Replace String(replace all?=TRUE ("replace all? (F)"), input string=w4191, search string="/") -> (result string=w4212:string)  [unwired: 5 in, 3 out]
                n1715 = for {
                  tunnel: [w4246] -> _ mode=indexing
                  tunnel: [w4251] -> w4224 mode=indexing
                  tunnel: w4225 -> [w4250] mode=indexing
                  tunnel: w4223 -> [w4246] mode=indexing
                  tunnel: w4222 -> [w4245] mode=indexing
                  tunnel: [w4246] -> w4221 mode=indexing
                  tunnel: [w4245] -> w4220 mode=indexing
                  tunnel: w4219 -> [w4240]
                  tunnel: w4218 -> [w4239]
                  tunnel: w4217 -> [w4238] mode=indexing
                  tunnel: w4216 -> [w4237]
                  tunnel: [w4231] -> w4215
                  tunnel: [w4231] -> w4214
                  n1716 = Join Numbers(hi=w4240, lo=w4239) -> ((hi.lo)=w4242:u32)
                  n1717 = To Double Precision Float(number=w4238) -> (double precision float=w4243:dbl)
                  n1718 = Number To Decimal String(number=w4250) -> (decimal integer string=w4249:string)  [unwired: 1 in]
                  n1719 = Number To Fractional String(number=w4246, precision (6)=i16 3 ("width (-)")) -> (F-format string=w4252:string)  [unwired: 2 in]
                  n1720 = Number To Fractional String(number=w4245, width (-)=i16 3) -> (F-format string=w4248:string)  [unwired: 2 in]
                  n1721 = Divide(x=w4243, y=w4237) -> (x/y=w4244:dbl)
                  n1722 = Build Array(w4249, w4252, w4248) -> (w4251:string[])
                  n1723 = To Unsigned Quad Integer(1:w4242) -> (0:w4241:u64)
                  n1724 = call "Unix Time to Timestamp.vi"("Fractional Second"=w4244, "Unix Time (s)"=w4241) -> ("Timestamp"=w4232:timestamp)  [unwired: 8 in, 1 out]
                  n1725 = Format Date/Time String(seconds (now)=w4232, UTC format=TRUE) -> (date/time string=w4233:string)  [unwired: 1 in]
                  n1726 = Scan From String(format string="%<%x %H:%M:%S%3u>T", input string=w4233) -> (output 1=w4234:timestamp)  [unwired: 3 in, 3 out]
                  n1727 = To Double Precision Float(number=w4234) -> (double precision float=w4231:dbl)
                }
                n1728 = Concatenate Strings(w4189, "TimeStamp;Measure Ch_X(g);INC_X(Deg);", "\n") -> (w4205:string)
                n1729 = Concatenate Strings(w4212, "_" ("string"), "S_E_T.csv") -> (w4213:string)
                n1730 = call <vilib>:"Get System Directory.vi"("system directory type"=w4196) -> ("system directory"=w4206:path)  [unwired: 10 in]
                n1731 = Build Path(base path=w4206, name or relative path="Logfile") -> (appended path=w4207:path)
                n1732 = call <vilib>:"Check if File or Folder Exists.vi"("path"=w4207) -> ("file or folder exists?"=w4208:bool, "dup path"=w4209:path)  [unwired: 8 in, 1 out]
                n1733 = case shown="False" w4208 {
                  tunnel: w4209 -> [w4229 w4230]
                  tunnel: [w4228 w4230] -> w4210
                  frame False {
                    n1734 = Create Folder(path (use dialog)=w4229) -> (created path=w4228:path)  [unwired: 2 in, 2 out]
                  }
                  frame True {
                  }
                }
                n1735 = Build Path(base path=w4210, name or relative path=w4213) -> (appended path=w4211:path)
                n1736 = Open/Create/Replace File(file path (use dialog)=w4211, operation (0:open)=T11."open or create") -> (refnum out=w4204:refnum<file>, error out=w4202:errorcluster)  [unwired: 4 in, 1 out]
                n1737 = Write to Text File(file (use dialog)=w4204, text=w4205, error in=w4202) -> (refnum out=w4203:refnum<file>, error out=w4201:errorcluster)  [unwired: 1 in, 1 out]
                n1738 = Close File(refnum=w4203, error in=w4201) -> (path=w4190:path)  [unwired: 1 out]
              }
              frame 11 {
                w4261 = T14 2 items=["User Home"=0, "User Desktop"=1, "User Documents"=2, "User Application Data"=3, "User Preferences"=4, "User Temporary"=5, "Public Documents"=6, "Public Application Data"=7, "Public Preferences"=8, "Public Cache"=13, "System Core Libraries"=9, "System Installed Libraries"=10, "Application Files"=11, "Boot Volume Root"=12] ("system directory type")
                n1739 = Search and Replace String(replace all?=TRUE ("replace all? (F)"), input string=w4256, search string="/") -> (result string=w4277:string)  [unwired: 5 in, 3 out]
                n1740 = Concatenate Strings(w4254, "TimeStamp;Measure Ch_Z(g);Ch_X(g);INC_X(Deg);", "\n") -> (w4270:string)
                n1741 = Concatenate Strings(w4277, "_" ("string"), "S_E_T.csv") -> (w4278:string)
                n1742 = call <vilib>:"Get System Directory.vi"("system directory type"=w4261) -> ("system directory"=w4271:path)  [unwired: 10 in]
                n1743 = Decimate 1D Array(w4294) -> (w4292:dbl[], w4291:dbl[], w4289:dbl[])
                n1744 = for {
                  tunnel: [w4322] -> w4290 mode=indexing
                  tunnel: w4293 -> [w4318] mode=indexing
                  tunnel: w4292 -> [w4315] mode=indexing
                  tunnel: w4291 -> [w4314] mode=indexing
                  tunnel: w4289 -> [w4313] mode=indexing
                  tunnel: [w4315] -> w4288 mode=indexing
                  tunnel: [w4314] -> w4287 mode=indexing
                  tunnel: [w4313] -> w4286 mode=indexing
                  tunnel: w4285 -> [w4308]
                  tunnel: w4284 -> [w4307]
                  tunnel: w4283 -> [w4306] mode=indexing
                  tunnel: w4282 -> [w4305]
                  tunnel: [w4299] -> w4281
                  tunnel: [w4299] -> w4280
                  tunnel: [w4299] -> w4279
                  n1745 = Join Numbers(hi=w4308, lo=w4307) -> ((hi.lo)=w4310:u32)
                  n1746 = To Double Precision Float(number=w4306) -> (double precision float=w4311:dbl)
                  n1747 = Number To Decimal String(number=w4318) -> (decimal integer string=w4321:string)  [unwired: 1 in]
                  n1748 = Number To Fractional String(number=w4315, precision (6)=i16 3 ("width (-)")) -> (F-format string=w4323:string)  [unwired: 2 in]
                  n1749 = Number To Fractional String(number=w4314, width (-)=i16 3) -> (F-format string=w4320:string)  [unwired: 2 in]
                  n1750 = Number To Fractional String(number=w4313, width (-)=i16 3) -> (F-format string=w4316:string)  [unwired: 2 in]
                  n1751 = Build Array(w4321, w4323, w4320, w4316) -> (w4322:string[])
                  n1752 = Divide(x=w4311, y=w4305) -> (x/y=w4312:dbl)
                  n1753 = To Unsigned Quad Integer(1:w4310) -> (0:w4309:u64)
                  n1754 = call "Unix Time to Timestamp.vi"("Fractional Second"=w4312, "Unix Time (s)"=w4309) -> ("Timestamp"=w4300:timestamp)  [unwired: 8 in, 1 out]
                  n1755 = Format Date/Time String(seconds (now)=w4300, UTC format=TRUE) -> (date/time string=w4301:string)  [unwired: 1 in]
                  n1756 = Scan From String(format string="%<%x %H:%M:%S%3u>T", input string=w4301) -> (output 1=w4302:timestamp)  [unwired: 3 in, 3 out]
                  n1757 = To Double Precision Float(number=w4302) -> (double precision float=w4299:dbl)
                }
                n1758 = Build Path(base path=w4271, name or relative path="Logfile") -> (appended path=w4272:path)
                n1759 = call <vilib>:"Check if File or Folder Exists.vi"("path"=w4272) -> ("file or folder exists?"=w4273:bool, "dup path"=w4274:path)  [unwired: 8 in, 1 out]
                n1760 = case shown="False" w4273 {
                  tunnel: w4274 -> [w4297 w4298]
                  tunnel: [w4296 w4298] -> w4275
                  frame False {
                    n1761 = Create Folder(path (use dialog)=w4297) -> (created path=w4296:path)  [unwired: 2 in, 2 out]
                  }
                  frame True {
                  }
                }
                n1762 = Build Path(base path=w4275, name or relative path=w4278) -> (appended path=w4276:path)
                n1763 = Open/Create/Replace File(file path (use dialog)=w4276, operation (0:open)=T11."open or create") -> (refnum out=w4269:refnum<file>, error out=w4267:errorcluster)  [unwired: 4 in, 1 out]
                n1764 = Write to Text File(file (use dialog)=w4269, text=w4270, error in=w4267) -> (refnum out=w4268:refnum<file>, error out=w4266:errorcluster)  [unwired: 1 in, 1 out]
                n1765 = Close File(refnum=w4268, error in=w4266) -> (path=w4255:path)  [unwired: 1 out]
              }
              frame 12 {
                w4332 = T14 2 items=["User Home"=0, "User Desktop"=1, "User Documents"=2, "User Application Data"=3, "User Preferences"=4, "User Temporary"=5, "Public Documents"=6, "Public Application Data"=7, "Public Preferences"=8, "Public Cache"=13, "System Core Libraries"=9, "System Installed Libraries"=10, "Application Files"=11, "Boot Volume Root"=12] ("system directory type")
                n1766 = Decimate 1D Array(w4362) -> (w4360:dbl[], w4359:dbl[])
                n1767 = Search and Replace String(replace all?=TRUE ("replace all? (F)"), input string=w4327, search string="/") -> (result string=w4348:string)  [unwired: 5 in, 3 out]
                n1768 = Concatenate Strings(w4325, "TimeStamp;Measure Ch_Y(g);INC_X(Deg);", "\n") -> (w4341:string)
                n1769 = for {
                  tunnel: [w4387] -> w4358 mode=indexing
                  tunnel: w4361 -> [w4383] mode=indexing
                  tunnel: w4360 -> [w4382] mode=indexing
                  tunnel: w4359 -> [w4381] mode=indexing
                  tunnel: [w4382] -> w4357 mode=indexing
                  tunnel: [w4381] -> w4356 mode=indexing
                  tunnel: w4355 -> [w4376]
                  tunnel: w4354 -> [w4375]
                  tunnel: w4353 -> [w4374] mode=indexing
                  tunnel: w4352 -> [w4373]
                  tunnel: [w4367] -> w4351
                  tunnel: [w4367] -> w4350
                  n1770 = Join Numbers(hi=w4376, lo=w4375) -> ((hi.lo)=w4378:u32)
                  n1771 = To Double Precision Float(number=w4374) -> (double precision float=w4379:dbl)
                  n1772 = Number To Decimal String(number=w4383) -> (decimal integer string=w4386:string)  [unwired: 1 in]
                  n1773 = Number To Fractional String(number=w4382, precision (6)=i16 3 ("width (-)")) -> (F-format string=w4388:string)  [unwired: 2 in]
                  n1774 = Number To Fractional String(number=w4381, width (-)=i16 3) -> (F-format string=w4385:string)  [unwired: 2 in]
                  n1775 = Divide(x=w4379, y=w4373) -> (x/y=w4380:dbl)
                  n1776 = Build Array(w4386, w4388, w4385) -> (w4387:string[])
                  n1777 = To Unsigned Quad Integer(1:w4378) -> (0:w4377:u64)
                  n1778 = call "Unix Time to Timestamp.vi"("Fractional Second"=w4380, "Unix Time (s)"=w4377) -> ("Timestamp"=w4368:timestamp)  [unwired: 8 in, 1 out]
                  n1779 = Format Date/Time String(seconds (now)=w4368, UTC format=TRUE) -> (date/time string=w4369:string)  [unwired: 1 in]
                  n1780 = Scan From String(format string="%<%x %H:%M:%S%3u>T", input string=w4369) -> (output 1=w4370:timestamp)  [unwired: 3 in, 3 out]
                  n1781 = To Double Precision Float(number=w4370) -> (double precision float=w4367:dbl)
                }
                n1782 = Concatenate Strings(w4348, "_" ("string"), "S_E_T.csv") -> (w4349:string)
                n1783 = call <vilib>:"Get System Directory.vi"("system directory type"=w4332) -> ("system directory"=w4342:path)  [unwired: 10 in]
                n1784 = Build Path(base path=w4342, name or relative path="Logfile") -> (appended path=w4343:path)
                n1785 = call <vilib>:"Check if File or Folder Exists.vi"("path"=w4343) -> ("file or folder exists?"=w4344:bool, "dup path"=w4345:path)  [unwired: 8 in, 1 out]
                n1786 = case shown="False" w4344 {
                  tunnel: w4345 -> [w4365 w4366]
                  tunnel: [w4364 w4366] -> w4346
                  frame False {
                    n1787 = Create Folder(path (use dialog)=w4365) -> (created path=w4364:path)  [unwired: 2 in, 2 out]
                  }
                  frame True {
                  }
                }
                n1788 = Build Path(base path=w4346, name or relative path=w4349) -> (appended path=w4347:path)
                n1789 = Open/Create/Replace File(file path (use dialog)=w4347, operation (0:open)=T11."open or create") -> (refnum out=w4340:refnum<file>, error out=w4338:errorcluster)  [unwired: 4 in, 1 out]
                n1790 = Write to Text File(file (use dialog)=w4340, text=w4341, error in=w4338) -> (refnum out=w4339:refnum<file>, error out=w4337:errorcluster)  [unwired: 1 in, 1 out]
                n1791 = Close File(refnum=w4339, error in=w4337) -> (path=w4326:path)  [unwired: 1 out]
              }
              frame 13 {
                w4397 = T14 2 items=["User Home"=0, "User Desktop"=1, "User Documents"=2, "User Application Data"=3, "User Preferences"=4, "User Temporary"=5, "Public Documents"=6, "Public Application Data"=7, "Public Preferences"=8, "Public Cache"=13, "System Core Libraries"=9, "System Installed Libraries"=10, "Application Files"=11, "Boot Volume Root"=12] ("system directory type")
                n1792 = Search and Replace String(replace all?=TRUE ("replace all? (F)"), input string=w4392, search string="/") -> (result string=w4413:string)  [unwired: 5 in, 3 out]
                n1793 = Concatenate Strings(w4390, "TimeStamp;Measure Ch_Z(g);Ch_Y(g);INC_X(Deg)", "\n") -> (w4406:string)
                n1794 = Concatenate Strings(w4413, "_" ("string"), "S_E_T.csv") -> (w4414:string)
                n1795 = call <vilib>:"Get System Directory.vi"("system directory type"=w4397) -> ("system directory"=w4407:path)  [unwired: 10 in]
                n1796 = Decimate 1D Array(w4430) -> (w4425:dbl[], w4428:dbl[], w4427:dbl[])
                n1797 = for {
                  tunnel: [w4458] -> w4426 mode=indexing
                  tunnel: w4429 -> [w4454] mode=indexing
                  tunnel: w4425 -> [w4453] mode=indexing
                  tunnel: w4428 -> [w4452] mode=indexing
                  tunnel: w4427 -> [w4451] mode=indexing
                  tunnel: [w4453] -> w4424 mode=indexing
                  tunnel: [w4452] -> w4423 mode=indexing
                  tunnel: [w4451] -> w4422 mode=indexing
                  tunnel: w4421 -> [w4446]
                  tunnel: w4420 -> [w4445]
                  tunnel: w4419 -> [w4444] mode=indexing
                  tunnel: w4418 -> [w4443]
                  tunnel: [w4435] -> w4417
                  tunnel: [w4435] -> w4416
                  tunnel: [w4435] -> w4415
                  n1798 = Join Numbers(hi=w4446, lo=w4445) -> ((hi.lo)=w4448:u32)
                  n1799 = To Double Precision Float(number=w4444) -> (double precision float=w4449:dbl)
                  n1800 = Number To Decimal String(number=w4454) -> (decimal integer string=w4457:string)  [unwired: 1 in]
                  n1801 = Number To Fractional String(number=w4453, precision (6)=i16 3 ("width (-)")) -> (F-format string=w4459:string)  [unwired: 2 in]
                  n1802 = Number To Fractional String(number=w4452, precision (6)=i16 3 ("width (-)")) -> (F-format string=w4456:string)  [unwired: 2 in]
                  n1803 = Number To Fractional String(number=w4451, precision (6)=i16 3 ("width (-)")) -> (F-format string=w4455:string)  [unwired: 2 in]
                  n1804 = Build Array(w4457, w4459, w4456, w4455) -> (w4458:string[])
                  n1805 = Divide(x=w4449, y=w4443) -> (x/y=w4450:dbl)
                  n1806 = To Unsigned Quad Integer(1:w4448) -> (0:w4447:u64)
                  n1807 = call "Unix Time to Timestamp.vi"("Fractional Second"=w4450, "Unix Time (s)"=w4447) -> ("Timestamp"=w4436:timestamp)  [unwired: 8 in, 1 out]
                  n1808 = Format Date/Time String(seconds (now)=w4436, UTC format=TRUE) -> (date/time string=w4437:string)  [unwired: 1 in]
                  n1809 = Scan From String(format string="%<%x %H:%M:%S%3u>T", input string=w4437) -> (output 1=w4438:timestamp)  [unwired: 3 in, 3 out]
                  n1810 = To Double Precision Float(number=w4438) -> (double precision float=w4435:dbl)
                }
                n1811 = Build Path(base path=w4407, name or relative path="Logfile") -> (appended path=w4408:path)
                n1812 = call <vilib>:"Check if File or Folder Exists.vi"("path"=w4408) -> ("file or folder exists?"=w4409:bool, "dup path"=w4410:path)  [unwired: 8 in, 1 out]
                n1813 = case shown="False" w4409 {
                  tunnel: w4410 -> [w4433 w4434]
                  tunnel: [w4432 w4434] -> w4411
                  frame False {
                    n1814 = Create Folder(path (use dialog)=w4433) -> (created path=w4432:path)  [unwired: 2 in, 2 out]
                  }
                  frame True {
                  }
                }
                n1815 = Build Path(base path=w4411, name or relative path=w4414) -> (appended path=w4412:path)
                n1816 = Open/Create/Replace File(file path (use dialog)=w4412, operation (0:open)=T11."open or create") -> (refnum out=w4405:refnum<file>, error out=w4403:errorcluster)  [unwired: 4 in, 1 out]
                n1817 = Write to Text File(file (use dialog)=w4405, text=w4406, error in=w4403) -> (refnum out=w4404:refnum<file>, error out=w4402:errorcluster)  [unwired: 1 in, 1 out]
                n1818 = Close File(refnum=w4404, error in=w4402) -> (path=w4391:path)  [unwired: 1 out]
              }
              frame 14 {
                w4468 = T14 2 items=["User Home"=0, "User Desktop"=1, "User Documents"=2, "User Application Data"=3, "User Preferences"=4, "User Temporary"=5, "Public Documents"=6, "Public Application Data"=7, "Public Preferences"=8, "Public Cache"=13, "System Core Libraries"=9, "System Installed Libraries"=10, "Application Files"=11, "Boot Volume Root"=12] ("system directory type")
                n1819 = Search and Replace String(replace all?=TRUE ("replace all? (F)"), input string=w4463, search string="/") -> (result string=w4484:string)  [unwired: 5 in, 3 out]
                n1820 = Concatenate Strings(w4461, "TimeStamp;Measure Ch_X(g);Ch_Y(g);INC_X(Deg)", "\n") -> (w4477:string)
                n1821 = Concatenate Strings(w4484, "_" ("string"), "S_E_T.csv") -> (w4485:string)
                n1822 = call <vilib>:"Get System Directory.vi"("system directory type"=w4468) -> ("system directory"=w4478:path)  [unwired: 10 in]
                n1823 = Decimate 1D Array(w4501) -> (w4499:dbl[], w4498:dbl[], w4497:dbl[])
                n1824 = for {
                  tunnel: [w4529] -> w4496 mode=indexing
                  tunnel: w4500 -> [w4525] mode=indexing
                  tunnel: w4499 -> [w4524] mode=indexing
                  tunnel: w4498 -> [w4523] mode=indexing
                  tunnel: w4497 -> [w4522] mode=indexing
                  tunnel: [w4524] -> w4495 mode=indexing
                  tunnel: [w4523] -> w4494 mode=indexing
                  tunnel: [w4522] -> w4493 mode=indexing
                  tunnel: w4492 -> [w4517]
                  tunnel: w4491 -> [w4516]
                  tunnel: w4490 -> [w4515] mode=indexing
                  tunnel: w4489 -> [w4514]
                  tunnel: [w4506] -> w4488
                  tunnel: [w4506] -> w4487
                  tunnel: [w4506] -> w4486
                  n1825 = Join Numbers(hi=w4517, lo=w4516) -> ((hi.lo)=w4519:u32)
                  n1826 = To Double Precision Float(number=w4515) -> (double precision float=w4520:dbl)
                  n1827 = Number To Decimal String(number=w4525) -> (decimal integer string=w4528:string)  [unwired: 1 in]
                  n1828 = Number To Fractional String(number=w4524, precision (6)=i16 3 ("width (-)")) -> (F-format string=w4530:string)  [unwired: 2 in]
                  n1829 = Number To Fractional String(number=w4523, precision (6)=i16 3 ("width (-)")) -> (F-format string=w4527:string)  [unwired: 2 in]
                  n1830 = Number To Fractional String(number=w4522, precision (6)=i16 3 ("width (-)")) -> (F-format string=w4526:string)  [unwired: 2 in]
                  n1831 = Build Array(w4528, w4530, w4527, w4526) -> (w4529:string[])
                  n1832 = Divide(x=w4520, y=w4514) -> (x/y=w4521:dbl)
                  n1833 = To Unsigned Quad Integer(1:w4519) -> (0:w4518:u64)
                  n1834 = call "Unix Time to Timestamp.vi"("Fractional Second"=w4521, "Unix Time (s)"=w4518) -> ("Timestamp"=w4507:timestamp)  [unwired: 8 in, 1 out]
                  n1835 = Format Date/Time String(seconds (now)=w4507, UTC format=TRUE) -> (date/time string=w4508:string)  [unwired: 1 in]
                  n1836 = Scan From String(format string="%<%x %H:%M:%S%3u>T", input string=w4508) -> (output 1=w4509:timestamp)  [unwired: 3 in, 3 out]
                  n1837 = To Double Precision Float(number=w4509) -> (double precision float=w4506:dbl)
                }
                n1838 = Build Path(base path=w4478, name or relative path="Logfile") -> (appended path=w4479:path)
                n1839 = call <vilib>:"Check if File or Folder Exists.vi"("path"=w4479) -> ("file or folder exists?"=w4480:bool, "dup path"=w4481:path)  [unwired: 8 in, 1 out]
                n1840 = case shown="False" w4480 {
                  tunnel: w4481 -> [w4504 w4505]
                  tunnel: [w4503 w4505] -> w4482
                  frame False {
                    n1841 = Create Folder(path (use dialog)=w4504) -> (created path=w4503:path)  [unwired: 2 in, 2 out]
                  }
                  frame True {
                  }
                }
                n1842 = Build Path(base path=w4482, name or relative path=w4485) -> (appended path=w4483:path)
                n1843 = Open/Create/Replace File(file path (use dialog)=w4483, operation (0:open)=T11."open or create") -> (refnum out=w4476:refnum<file>, error out=w4474:errorcluster)  [unwired: 4 in, 1 out]
                n1844 = Write to Text File(file (use dialog)=w4476, text=w4477, error in=w4474) -> (refnum out=w4475:refnum<file>, error out=w4473:errorcluster)  [unwired: 1 in, 1 out]
                n1845 = Close File(refnum=w4475, error in=w4473) -> (path=w4462:path)  [unwired: 1 out]
              }
              frame 15 {
                w4539 = T14 2 items=["User Home"=0, "User Desktop"=1, "User Documents"=2, "User Application Data"=3, "User Preferences"=4, "User Temporary"=5, "Public Documents"=6, "Public Application Data"=7, "Public Preferences"=8, "Public Cache"=13, "System Core Libraries"=9, "System Installed Libraries"=10, "Application Files"=11, "Boot Volume Root"=12] ("system directory type")
                n1846 = Search and Replace String(replace all?=TRUE ("replace all? (F)"), input string=w4534, search string="/") -> (result string=w4555:string)  [unwired: 5 in, 3 out]
                n1847 = Concatenate Strings(w4532, "TimeStamp;MeasureCh_Z(g);Ch_X(g);Ch_Y(g);INC_X(Deg)", "\n") -> (w4548:string)
                n1848 = Concatenate Strings(w4555, "_" ("string"), "S_E_T.csv") -> (w4556:string)
                n1849 = call <vilib>:"Get System Directory.vi"("system directory type"=w4539) -> ("system directory"=w4549:path)  [unwired: 10 in]
                n1850 = Decimate 1D Array(w4575) -> (w4573:dbl[], w4572:dbl[], w4571:dbl[], w4569:dbl[])
                n1851 = for {
                  tunnel: [w4606] -> w4570 mode=indexing
                  tunnel: w4574 -> [w4601] mode=indexing
                  tunnel: w4573 -> [w4600] mode=indexing
                  tunnel: w4572 -> [w4599] mode=indexing
                  tunnel: w4571 -> [w4598] mode=indexing
                  tunnel: w4569 -> [w4597] mode=indexing
                  tunnel: [w4600] -> w4568 mode=indexing
                  tunnel: [w4599] -> w4567 mode=indexing
                  tunnel: [w4598] -> w4566 mode=indexing
                  tunnel: [w4597] -> w4565 mode=indexing
                  tunnel: w4564 -> [w4592]
                  tunnel: w4563 -> [w4591]
                  tunnel: w4562 -> [w4590] mode=indexing
                  tunnel: w4561 -> [w4589]
                  tunnel: [w4580] -> w4560
                  tunnel: [w4580] -> w4559
                  tunnel: [w4580] -> w4558
                  tunnel: [w4580] -> w4557
                  n1852 = Join Numbers(hi=w4592, lo=w4591) -> ((hi.lo)=w4594:u32)
                  n1853 = To Double Precision Float(number=w4590) -> (double precision float=w4595:dbl)
                  n1854 = Number To Decimal String(number=w4601) -> (decimal integer string=w4605:string)  [unwired: 1 in]
                  n1855 = Number To Fractional String(number=w4600, precision (6)=i16 3 ("width (-)")) -> (F-format string=w4607:string)  [unwired: 2 in]
                  n1856 = Number To Fractional String(number=w4599, precision (6)=i16 3 ("width (-)")) -> (F-format string=w4604:string)  [unwired: 2 in]
                  n1857 = Number To Fractional String(number=w4598, precision (6)=i16 3 ("width (-)")) -> (F-format string=w4603:string)  [unwired: 2 in]
                  n1858 = Number To Fractional String(number=w4597, precision (6)=i16 3 ("width (-)")) -> (F-format string=w4602:string)  [unwired: 2 in]
                  n1859 = Build Array(w4605, w4607, w4604, w4603, w4602) -> (w4606:string[])
                  n1860 = Divide(x=w4595, y=w4589) -> (x/y=w4596:dbl)
                  n1861 = To Unsigned Quad Integer(1:w4594) -> (0:w4593:u64)
                  n1862 = call "Unix Time to Timestamp.vi"("Fractional Second"=w4596, "Unix Time (s)"=w4593) -> ("Timestamp"=w4581:timestamp)  [unwired: 8 in, 1 out]
                  n1863 = Format Date/Time String(seconds (now)=w4581, UTC format=TRUE) -> (date/time string=w4582:string)  [unwired: 1 in]
                  n1864 = Scan From String(format string="%<%x %H:%M:%S%3u>T", input string=w4582) -> (output 1=w4583:timestamp)  [unwired: 3 in, 3 out]
                  n1865 = To Double Precision Float(number=w4583) -> (double precision float=w4580:dbl)
                }
                n1866 = Build Path(base path=w4549, name or relative path="Logfile") -> (appended path=w4550:path)
                n1867 = call <vilib>:"Check if File or Folder Exists.vi"("path"=w4550) -> ("file or folder exists?"=w4551:bool, "dup path"=w4552:path)  [unwired: 8 in, 1 out]
                n1868 = case shown="False" w4551 {
                  tunnel: w4552 -> [w4578 w4579]
                  tunnel: [w4577 w4579] -> w4553
                  frame False {
                    n1869 = Create Folder(path (use dialog)=w4578) -> (created path=w4577:path)  [unwired: 2 in, 2 out]
                  }
                  frame True {
                  }
                }
                n1870 = Build Path(base path=w4553, name or relative path=w4556) -> (appended path=w4554:path)
                n1871 = Open/Create/Replace File(file path (use dialog)=w4554, operation (0:open)=T11."open or create") -> (refnum out=w4547:refnum<file>, error out=w4545:errorcluster)  [unwired: 4 in, 1 out]
                n1872 = Write to Text File(file (use dialog)=w4547, text=w4548, error in=w4545) -> (refnum out=w4546:refnum<file>, error out=w4544:errorcluster)  [unwired: 1 in, 1 out]
